vi "calculateColorMode.vi"(0 "Camera in":refnum<class "Camera.lvclass">, 5 "roi":cluster{"x0":u64, "y0":u64, "x1":u64, "y1":u64}, 11 "error in (no error)":errorcluster) -> (4 "Camera out":refnum<class "Camera.lvclass">, 6 "colorMode":i32, 15 "error out":errorcluster)   [LabVIEW 2019, in "Camera.lvclass"]
doc: "Retreive the rec handle.\nThis handle allows direct access to all underlying functions of the pco.recorder."
uses:
  Camera.lvclass
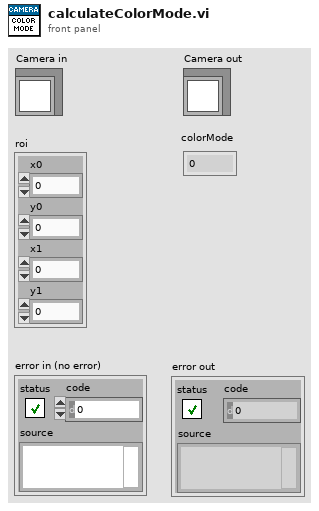
[diagram p1: front panel]
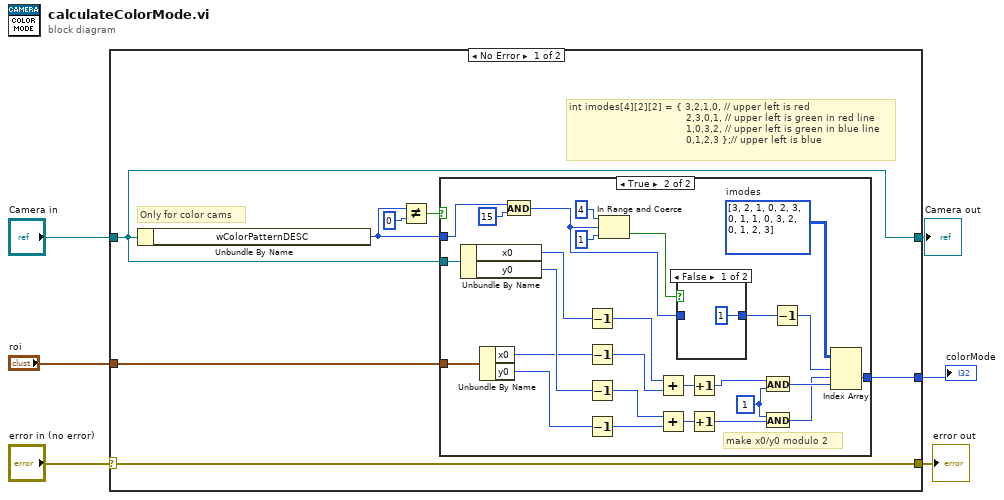
[diagram p0: block diagram]
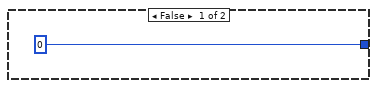
[diagram p2: hidden frame]
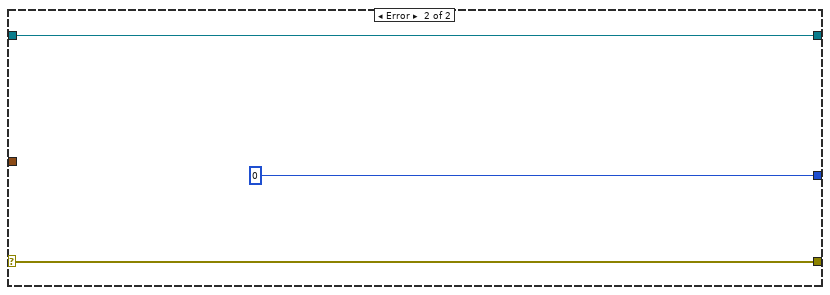
[diagram p4: hidden frame]
diagram:
  n1 = case shown="No Error" "error in (no error)" {
    selector: "error in (no error)" -> [w13 w46]
    tunnel: [w13 w46] -> w4
    tunnel: [w8 w45] -> w5
    tunnel: "Camera in" -> [w8 w45]
    tunnel: "roi" -> [w9 _]
    tunnel: [w7 0] -> w1
    frame No Error {
      # "int imodes[4][2][2] = { 3,2,1,0, // upper left is red\n                                       2,3,0,1, // upper left is green in red line\n                                       1,0,3,2, // upper left is green in blue line\n                                       0,1,2,3 };// upper left is blue"
      # "Only for color cams"
      n2 = Unbundle By Name(w8) -> ("wColorPatternDESC"=w10:u16)
      n3 = Not Equal?(x=w10, y=u16 0) -> (x != y?=w11:bool)
      n4 = case shown="True" w11 {
        tunnel: w10 -> [_ w29]
        tunnel: w9 -> [_ w41]
        tunnel: w8 -> [_ w40]
        tunnel: [0 w20] -> w7
        frame False {
        }
        frame True {
          w16 = u64 1 ("y")
          w21 = i32[][][] [[[3, 2], [1, 0]], [[2, 3], [0, 1]], [[1, 0], [3, 2]], [[0, 1], [2, 3]]]  # imodes
          # "make x0/y0 modulo 2"
          n5 = Unbundle By Name(w40) -> ("x0"=w39:u64, "y0"=w38:u64)
          n6 = Unbundle By Name(w41) -> ("x0"=w37:u64, "y0"=w36:u64)
          n7 = And(x=w29, y=u16 15) -> (x .and. y?=w24:u16)
          n8 = Decrement(x=w39) -> (x-1=w35:u64)
          n9 = Decrement(x=w37) -> (x-1=w34:u64)
          n10 = Decrement(x=w38) -> (x-1=w33:u64)
          n11 = Decrement(x=w36) -> (x-1=w32:u64)
          n12 = In Range and Coerce(upper limit=u16 4, x=w24, lower limit=u16 1) -> (In Range?=w25:bool)  [unwired: 1 out]
          n13 = Add(x=w35, y=w34) -> (x+y=w31:u64)
          n14 = Add(x=w33, y=w32) -> (x+y=w30:u64)
          n15 = case shown="False" w25 {
            tunnel: w24 -> [_ w43]
            tunnel: [u16 1 ("lower limit") w43] -> w23
            frame False {
            }
            frame True {
            }
          }
          n16 = Increment(x=w31) -> (x+1=w19:u64)
          n17 = Increment(x=w30) -> (x+1=w17:u64)
          n18 = And(x=w19, y=w16) -> (x .and. y?=w18:u64)
          n19 = And(x=w16, y=w17) -> (x .and. y?=w15:u64)
          n20 = Decrement(x=w23) -> (x-1=w22:u16)
          n21 = Index Array(array=w21, index (dim 0)=w22, index (dim 1)=w15, index (dim 2)=w18) -> (element=w20:i32)
        }
      }
    }
    frame Error {
    }
  }
  "error out" <- w4
  "Camera out" <- w5
  "colorMode" <- w1
